vi "Sequence Experiment.Client.vi"(8 "error in (no error)":errorcluster, 9 "Data":variant, 10 "Command":T1, 11 "Sequence Experiment":refnum<class "Sequence Experiment.lvclass">) -> (0 "error out":errorcluster, 1 "Data out":variant, 2 "Command":string, 3 "Sequence Experiment out":refnum<class "Sequence Experiment.lvclass">)   [LabVIEW 2019, in "Sequence Experiment.lvclass"]
uses:
  Sequence Experiment.lvclass
  5a5600e7-4988-4326-8f4e-678d31c4f83a.vi
  Typedefs/Sequence Experiment.Commands--Enum.ctl
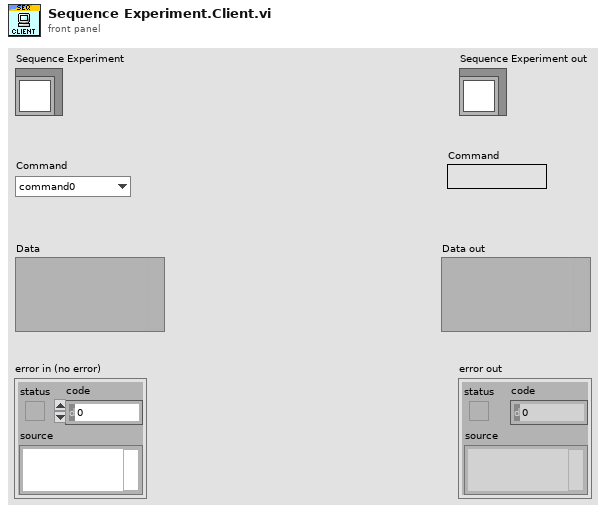
[diagram p1: front panel]
types:
  T1 = typedef "Sequence Experiment.lvclass/Sequence Experiment.Commands--Enum.ctl" = enum16{"command0", "command1", "command2"}
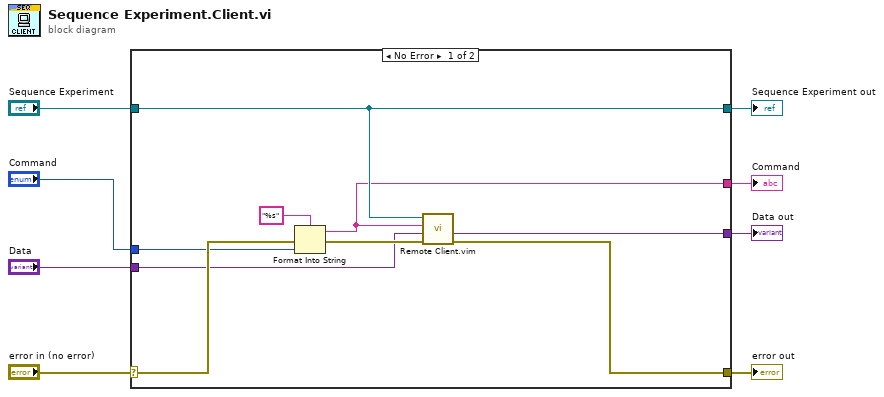
[diagram p0: block diagram]
diagram:
  n1 = case shown="No Error" "error in (no error)" {
    selector: "error in (no error)" -> [w14 w19]
    tunnel: [w13 w19] -> w7
    tunnel: [w17 w18] -> w5
    tunnel: "Sequence Experiment" -> [w17 w18]
    tunnel: "Data" -> [w9 _]
    tunnel: "Command" -> [w12 _]
    tunnel: [w11 _] -> w2
    tunnel: [w10 _] -> w1
    frame No Error {
      n2 = Format Into String(format string="%s", error in=w14, w12) -> (resulting string=w10:string, error out=w15:errorcluster)  [unwired: 1 in]
      n3 = call "Remote Client.vim"("error in (no error)"=w15, "params"=w9, "method"=w10, "Instrument in"=w17) -> ("error out"=w13:errorcluster, "Data out"=w11:variant)  [unwired: 4 in, 2 out]
    }
    frame Error {
    }
  }
  "error out" <- w7
  "Sequence Experiment out" <- w5
  "Data out" <- w2
  "Command" <- w1
